vi "subsystem_logEvent_Heartbeat.vi"(8 "error in (no error)":errorcluster, 10 "logevent_Heartbeat in":T1, 11 "ProgrammaticInitialization in":refnum<class "ProgrammaticInitialization.lvclass">) -> (0 "error out":errorcluster, 2 "logevent_Heartbeat":T1, 3 "ProgrammaticInitialization out":refnum<class "ProgrammaticInitialization.lvclass">)   [LabVIEW 2016, in "ProgrammaticInitialization.lvclass"]
uses:
  ProgrammaticInitialization.lvclass
  ts_sallv_sedspectrometer/DataTypes/logevent_Heartbeat.ctl
  ts_sallv_sedspectrometer/SALLV_sedSpectrometer.lvlib
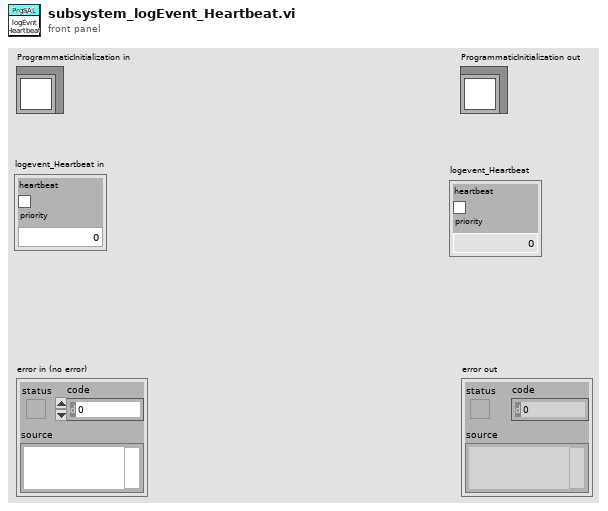
[diagram p1: front panel]
types:
  T1 = typedef "SALLV_sedSpectrometer.lvlib/logevent_Heartbeat.ctl" = cluster{"heartbeat":bool, "priority":i32}
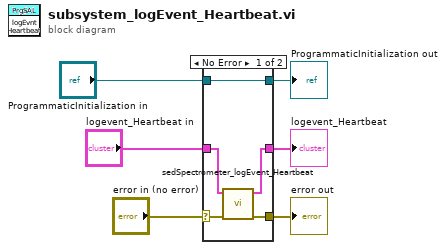
[diagram p0: block diagram]
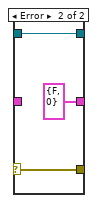
[diagram p2: hidden frame]
diagram:
  n1 = case shown="No Error" "error in (no error)" {
    selector: "error in (no error)" -> [w10 w14]
    tunnel: [w7 w14] -> w5
    tunnel: [w9 w13] -> w3
    tunnel: "ProgrammaticInitialization in" -> [w9 w13]
    tunnel: [w8 T1 {"heartbeat"=FALSE, "priority"=0} ("logevent_Heartbeat_Ctl out")] -> w2
    tunnel: "logevent_Heartbeat in" -> [w11 _]
    frame No Error {
      n2 = call "sedSpectrometer_logEvent_Heartbeat.vi"("error in (no error)"=w10, "logevent_Heartbeat_Ctl"=w11) -> ("error out"=w7:errorcluster, "logevent_Heartbeat_Ctl out"=w8:T1)  [unwired: 7 in, 1 out]
    }
    frame Error {
    }
  }
  "error out" <- w5
  "ProgrammaticInitialization out" <- w3
  "logevent_Heartbeat" <- w2
